vi "Test Upsampling.vi"() -> ()   [LabVIEW 2015]
uses:
  Utility VIs/Math VIs/LinSpace (x0-dx-npts).vi
  Utility VIs/Conversion VIs/Create Waveform Cluster (1D).vi
  <vilib>/Analysis/2dsp.llb/Rational Resample (single channel, DBL).vi
  <vilib>/Analysis/NI_AALPro.lvlib
panel:
  in  "Desired Fs":dbl format="%#_16g"
  out "Waveform Graph":cluster{dbl, "dx":dbl, "Y":dbl[]}[](graph)
  in  "T":dbl format="%#_16g"
  in  "Fs TDT":dbl format="%#_16g"
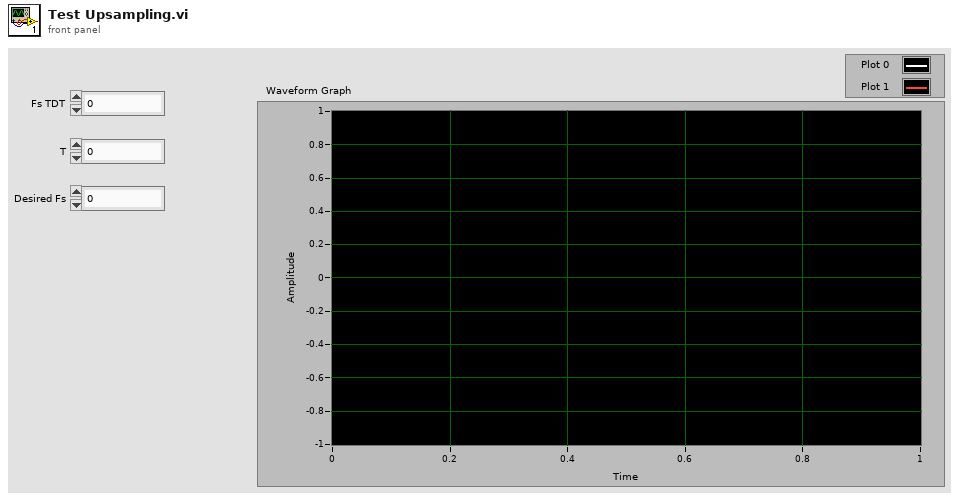
[diagram p1: front panel]
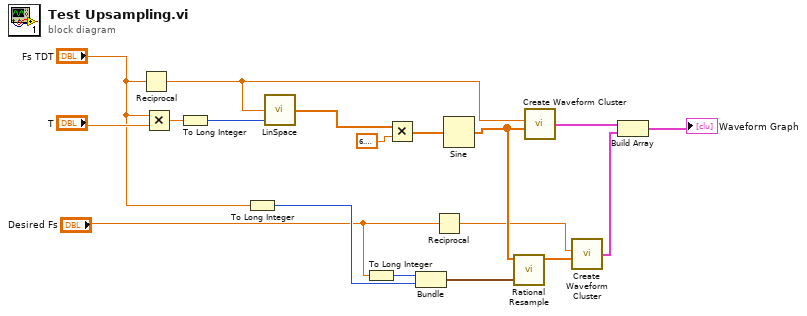
[diagram p0: block diagram]
diagram:
  n1 = Reciprocal(x="Fs TDT") -> (1/x=w5:dbl)
  n2 = Multiply(x="Fs TDT", y="T") -> (x*y=w17:dbl)
  n3 = To Long Integer(number=w17) -> (32bit integer=w16:i32)
  n4 = To Long Integer(number="Fs TDT") -> (32bit integer=w3:i32)
  n5 = call-poly "LinSpace.vi"("npts"=w16, "dx"=w5) -> ("Array"=w15:dbl[])  [unwired: 2 in, 1 out]
  n6 = To Long Integer(number="Desired Fs") -> (32bit integer=w2:i32)
  n7 = Multiply(x=w15, y=6.283185307179586) -> (x*y=w13:dbl[])
  n8 = Bundle(w2, w3) -> (w11:cluster{i32, i32})  [unwired: 1 in]
  n9 = Reciprocal(x="Desired Fs") -> (1/x=w4:dbl)
  n10 = Sine(x=w13) -> (sin(x)=w10:dbl[])
  n11 = call-poly <vilib>:"Rational Resample.vi"("resample factor"=w11, "X"=w10) -> ("Y"=w9:dbl[])  [unwired: 7 in, 2 out]
  n12 = call-poly "Create Waveform Cluster.vi"("dx"=w5, "Y"=w10) -> ("waveform cluster"=w12:cluster{dbl, "dx":dbl, "Y":dbl[]})  [unwired: 3 in]
  n13 = call-poly "Create Waveform Cluster.vi"("dx"=w4, "Y"=w9) -> ("waveform cluster"=w7:cluster{dbl, "dx":dbl, "Y":dbl[]})  [unwired: 3 in]
  n14 = Build Array(w12, w7) -> (→"Waveform Graph":cluster{dbl, "dx":dbl, "Y":dbl[]}[])
